vi "GenNewTraj.vi"(8 "Stoopid Overlap %":dbl min=0.0, 10 "Parameters":T4={"Sample Period (s)"=0.0, "Limits"={"Velocity (fps)"=6.0, "Accel (fps^2)"=15.0, "Jerk (fps^3)"=150.0, "StoopidFast (fps)"=6.0}, "Conditions"={"vInitial (fps)"=0.0, "vFinal (fps)"=0.0}, "Overrides"=[]} {"Overrides"."Angular Multiplier 2" step=5.0; "Overrides"."Angular Multiplier" step=5.0; "Limits"."StoopidFast (fps)" min=0.0; "Limits"."Jerk (fps^3)" min=0.0 step=1.0; "Limits"."Accel (fps^2)" min=0.0; "Limits"."Velocity (fps)" min=0.0}, 11 "Points in":cluster{"x":dbl, "y":dbl, "th":dbl}[](array[cluster])) -> (0 "Time & Dist":cluster{"Time (s)":dbl, "Distance (ft)":dbl}, 1 "Valid":bool, 2 "Trajectory Data":T1, 3 "Updated Waypoints":cluster{"x":dbl, "y":dbl, "th":dbl}[](array[cluster]))   [LabVIEW 2019]
uses:
  Types/Limits.ctl
  Types/Trajectory Data.ctl
  Types/Segment Type.ctl
  5b132355-d611-49ac-9db4-4ea5228ca0e8.vi
  Global Settings.vi
  Bezier/Generate Bezier Trajectory.vi
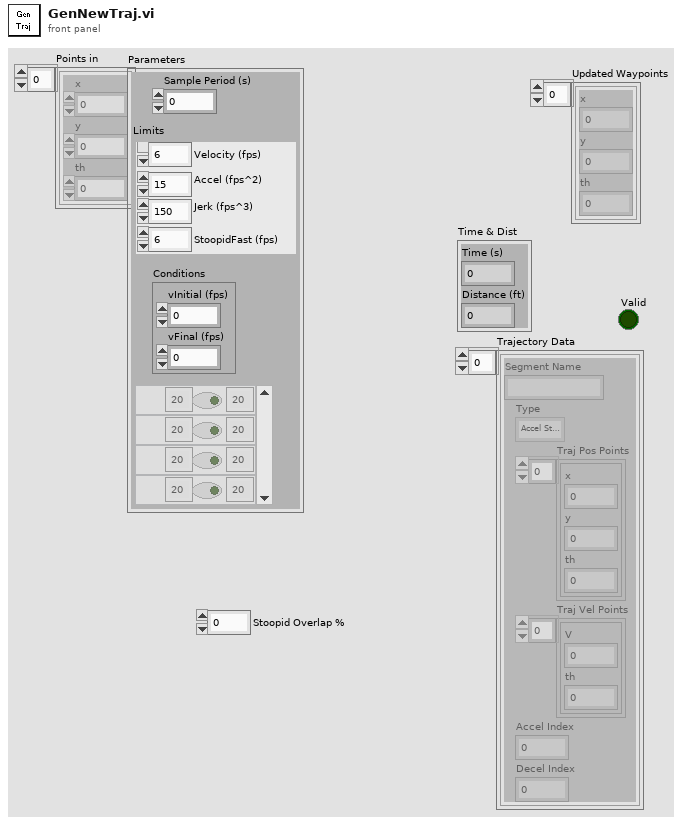
[diagram p1: front panel]
types:
  T1 = typedef "Trajectory Data.ctl" = cluster{"Segment Name":string, "Type":T2, "Traj Pos Points":cluster{"x":dbl, "y":dbl, "th":dbl}[], "Traj Vel Points":cluster{"V":dbl, "th":dbl}[], "Accel Index":i32, "Decel Index":i32}[]
  T2 = typedef "Segment Type.ctl" = enum16{"Accel Straight", "Const Straight", "Blend", "Circle", "Bezier"}
  T3 = typedef "Limits.ctl" = cluster{"Velocity (fps)":dbl, "Accel (fps^2)":dbl, "Jerk (fps^3)":dbl, "StoopidFast (fps)":dbl}
  T4 = cluster{"Sample Period (s)":dbl, "Limits":T3, "Conditions":cluster{"vInitial (fps)":dbl, "vFinal (fps)":dbl}, "Overrides":cluster{"Count":string, "Angular Multiplier":dbl, "1":bool, "Angular Multiplier 2":dbl}[]}
  T5 = cluster{"vInitial (fps)":dbl, "vFinal (fps)":dbl}
  T6 = cluster{"Count":string, "Angular Multiplier":dbl, "1":bool, "Angular Multiplier 2":dbl}[]
  T7 = typedef "Path Type.ctl" = enum16{"Clothoid", "Bezier"}
  T8 = cluster{"Path Type":T7, "Points in":cluster{"x":dbl, "y":dbl, "th":dbl}[], "Sample Period (s)":dbl, "Limits":T3, "Conditions":cluster{"vInitial (fps)":dbl, "vFinal (fps)":dbl}, "Overrides":cluster{"Count":string, "Angular Multiplier":dbl, "1":bool, "Angular Multiplier 2":dbl}[]}
  T9 = cluster{"Segment Name":string, "Type":enum16{"Accel Straight", "Const Straight", "Blend", "Circle"}, "Traj Pos Points":cluster{"x":dbl, "y":dbl, "th":dbl}[], "Traj Vel Points":cluster{"V":dbl, "th":dbl}[], "Accel Index":i32, "Decel Index":i32}[]
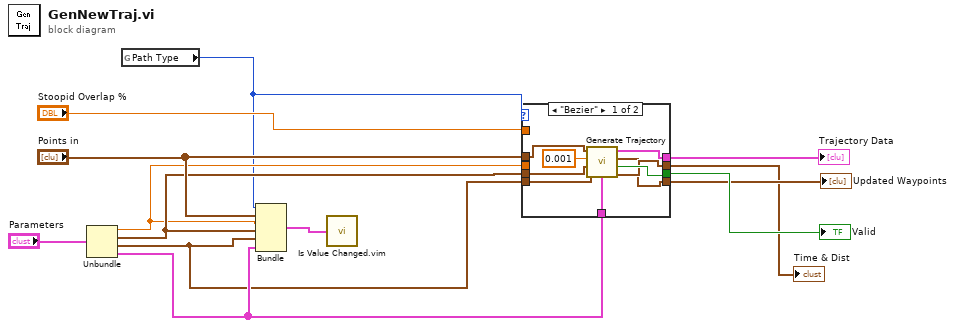
[diagram p0: block diagram]
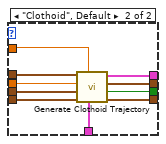
[diagram p2: hidden frame]
diagram:
  n1 = Unbundle("Parameters") -> ("Sample Period (s)"=w3:dbl, "Limits"=w6:T3, "Conditions"=w5:T5, "Overrides"=w8:T6)
  n2 = global read "Global Settings.vi" "Path Type"() -> (w2:T7)
  n3 = Bundle("Path Type"=w2, "Points in"="Points in", "Sample Period (s)"=w3, "Limits"=w6, "Conditions"=w5, "Overrides"=w8) -> (w9:T8)  [unwired: 1 in]
  n4 = call "Is Value Changed.vim"("value"=w9) -> ()  [unwired: 1 out]
  n5 = case shown="\"Bezier\"" w2 {
    tunnel: [w17 w32] -> w13
    tunnel: [w15 w31] -> w4
    tunnel: w5 -> [w19 w30]
    tunnel: w6 -> [w20 w29]
    tunnel: w8 -> [w18 w28]
    tunnel: [w14 w27] -> w12
    tunnel: [w16 w26] -> w1
    tunnel: "Stoopid Overlap %" -> [_ w25]
    tunnel: "Points in" -> [w21 w24]
    tunnel: w3 -> [_ w23]
    frame "Bezier" {
      n6 = call-poly "Generate Trajectory.vi"("Overrides"=w18, "Conditions"=w19, "Limits"=w20, "percision"=0.001, "WayPoints"=w21) -> ("Time & Dist"=w15:cluster{"Time (s)":dbl, "Distance (ft)":dbl}, "Valid"=w17:bool, "Updated Waypoints"=w14:cluster{"x":dbl, "y":dbl, "th":dbl}[], "Trajectory Data"=w16:T1)  [unwired: 3 in]
    }
    frame "Clothoid", Default {
      n7 = call "Generate Clothoid Trajectory.vi"("Overrides"=w28, "Stoopid Overlap %"=w25, "Conditions"=w30, "Limits"=w29, "Sample Period (s)"=w23, "WayPoints"=w24) -> ("Updated Waypoints"=w27:cluster{"x":dbl, "y":dbl, "th":dbl}[], "Valid"=w32:bool, "Time & Dist"=w31:cluster{"Time (s)":dbl, "Distance (ft)":dbl}, "Trajectory Data"=w26:T9)  [unwired: 2 in]
    }
  }
  "Valid" <- w13
  "Updated Waypoints" <- w12
  "Time & Dist" <- w4
  "Trajectory Data" <- w1
